vi "Process Guardian Go-NoGo Reply.vi"(8 "error in (no error)":errorcluster, 10 "Go-NoGo":T1, 11 "Tamer in":refnum<class "Tamer.lvclass">) -> (0 "error out":errorcluster, 3 "Tamer out":refnum<class "Tamer.lvclass">)   [LabVIEW 2020, in "TALOS.lvlib" / "Tamer.lvlib" / "Tamer.lvclass"]
uses:
  Tamer.lvclass
  C:/LabVIEW Code/TALOS/talos/Father of all uServices/Father of all uServices/Father of all uServices.lvclass
  Support VIs/Go-NoGo.ctl
  Reply.ctl
  Tamer.lvclass/Tamer.ctl
  Ancestor/Ancestor/Ancestor.lvclass/Ancestor.ctl
  FGV/Error Memory/Get Error Description.vi
  Support VIs/Get PC name.vi
  Ancestor/Ancestor/Read ID.vi
  Support VIs/Get Class Name.vi
  <vilib>/Utility/error.llb/Clear Errors.vi
  FGV/Error Memory/Error Memory Core.vi
  <vilib>/AdvancedString/Delimited String to 1D String Array.vi
  Support VIs/Circus Root Path.vi
  FGV/Error Memory/Error Crt Lvl checker.vi
  FGV/Error Memory/Error Memory Core.vi/40c8088d-b597-4017-91af-faa98e00292e.vi
  FGV/Error Memory/Error Memory Core.vi/d4a3ab98-063c-4e44-b43d-fbdcfe6c2be2.vi
  Support VIs/Global Memory.vi
  <vilib>/Utility/LVClass/Get LV Class Name.vi
  Support VIs/Is in Packed Library.vi
  Support VIs/TALOS Root path.vi
  Support VIs/Read CSV worksheet.vi
  Support VIs/Global Constants.vi
  <vilib>/Utility/error.llb/General Error Handler.vi
  Ancestor/Ancestor/Ancestor.lvclass
  <vilib>/Comparison/Equal/Equal Functor/Equal Functor.lvclass
  Father of all uServices/Father of all uServices/Father of all uServices.lvclass
  TALOS.lvlib
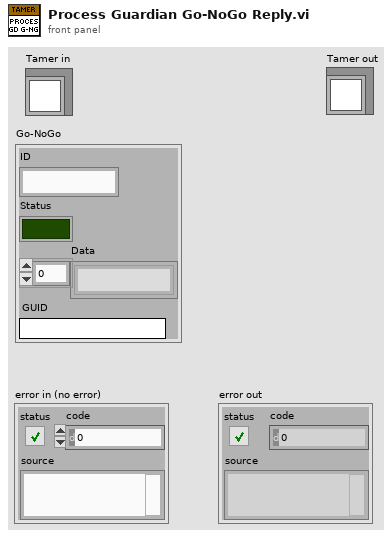
[diagram p1: front panel]
types:
  T1 = typedef "TALOS.lvlib/Go-NoGo.ctl" = cluster{"ID":string, "Status":bool, "Data":string[], "GUID":string}
  T2 = typedef "TALOS.lvlib/Tamer.lvlib/Tamer.lvclass/Reply.ctl" = cluster{"ID":string, "Status":bool, "GUID":string}
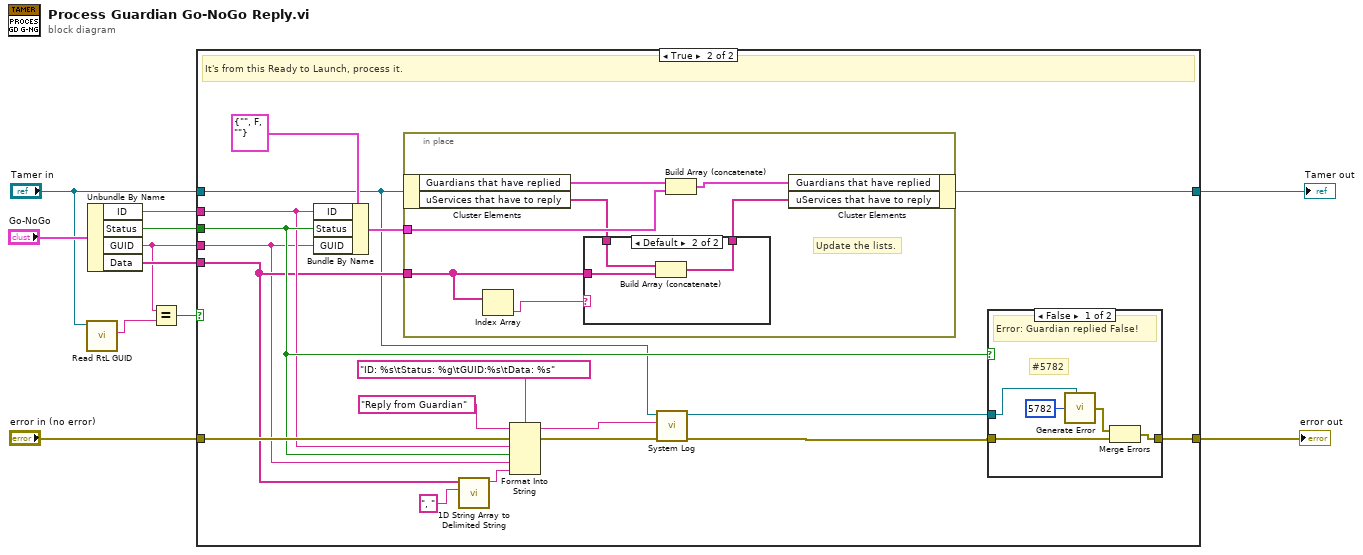
[diagram p0: block diagram]
diagram:
  n1 = call-dynamic "Read RtL GUID.vi"("Monkey in"="Tamer in") -> ("RtL GUID"=w3:string)  [unwired: 8 in, 2 out]
  n2 = Unbundle By Name("Go-NoGo") -> ("ID"=w6:string, "Status"=w9:bool, "GUID"=w2:string, "Data"=w5:string[])
  n3 = Equal?(x=w2, y=w3) -> (x = y?=w1:bool)
  n4 = case shown="True" w1 {
    tunnel: "error in (no error)" -> [w12 w31]
    tunnel: [w12 w23] -> w10
    tunnel: w9 -> [_ w22]
    tunnel: [w13 w21] -> w8
    tunnel: w6 -> [_ w19]
    tunnel: w5 -> [_ w18]
    tunnel: "Tamer in" -> [w13 w17]
    tunnel: w2 -> [_ w16]
    frame False {
      # "It's from a previous Ready to Launch, disregard it."
    }
    frame True {
      # "It's from this Ready to Launch, process it."
      n5 = Bundle By Name(cluster=T2 {"ID"="", "Status"=FALSE, "GUID"=""} ("Reply"), "ID"=w19, "Status"=w22, "GUID"=w16) -> (w24:T2)
      n6 = in-place {
        in-place-border: w24 -> [w43]
        in-place-border: w18 -> [w40]
        # "Update the lists."
        n7 = in-place-cluster #1(w17) -> ("Guardians that have replied"=w44:T2[], "uServices that have to reply"=w42:string[])
        n8 = Index Array(array=w40) -> (element=w39:string)  [unwired: 1 in]
        n9 = case shown="Default" w39 {
          tunnel: w42 -> [w45 w48]
          tunnel: w40 -> [_ w47]
          tunnel: [w45 w46] -> w41
          frame "PXI" {
            # "The PXI system don't have uServices!"
          }
          frame Default {
            n10 = Build Array (concatenate)(w48, w47) -> (w46:string[])
          }
        }
        n11 = Build Array (concatenate)(w44, w43) -> (w38:T2[])
        n12 = in-place-cluster #1("Guardians that have replied"=w38, "uServices that have to reply"=w41) -> (w21:refnum<class "Tamer.lvclass">)
      }
      n13 = call <vilib>:"1D String Array to Delimited String.vi"("delimiter"=", ", "string array"=w18) -> ("delimited string"=w20:string)  [unwired: 9 in]
      n14 = Format Into String(format string="ID: %s\tStatus: %g\tGUID:%s\tData: %s", initial string="Reply from Guardian", error in=w31, w19, w22, w16, w20) -> (resulting string=w28:string, error out=w27:errorcluster)
      n15 = call "System Log.vi"("error in (no error)"=w27, "Text to log"=w28, "uService Template in"=w17) -> ("error out"=w14:errorcluster, "uService Template out"=w15:refnum<class "Tamer.lvclass">)  [unwired: 7 in]
      n16 = case shown="False" w22 {
        tunnel: w14 -> [w36 w37]
        tunnel: [w35 w37] -> w23
        tunnel: w15 -> [w34 _]
        frame False {
          # "#5782"
          # "Error: Guardian replied False!"
          n17 = call "Generate Error.vi"("Class"=w34, "Error Code"=5782) -> ("error out"=w33:errorcluster)  [unwired: 5 in]
          n18 = Merge Errors(w33, w36) -> (w35:errorcluster)
        }
        frame True {
          # "All OK"
        }
      }
    }
  }
  "error out" <- w10
  "Tamer out" <- w8
